vi "Define_Indicies_for_Subtracks_Cost_F()-2.vi"(2 "[IN] Number of Rows":i32, 3 "[IN] Current index":i32, 4 "[IN] Subtracks":T1(array[cluster])) -> (0 "[OUT] Column \n# for Subtrack":i32, 1 "[OUT] Row # \nfor Subtrack":i32)   [LabVIEW 2013]
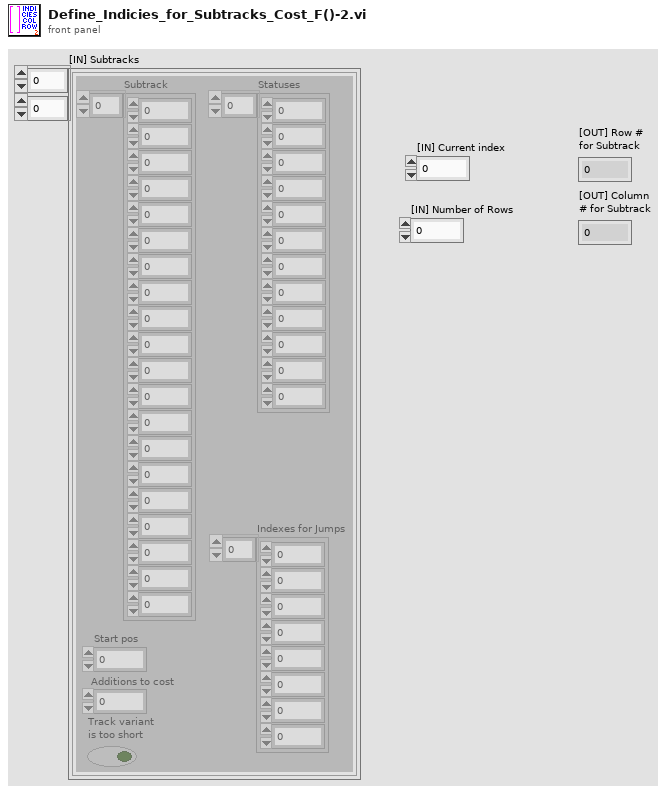
[diagram p1: front panel]
types:
  T1 = cluster{"Subtrack":dbl[], "Statuses":i16[], "Start pos":i32, "Additions to cost":i32, "Track variant \nis too short":bool, "Indexes for Jumps":i32[]}[][]
  T2 = cluster{"Subtrack":dbl[], "Statuses":i16[], "Start pos":i32, "Additions to cost":i32, "Track variant \nis too short":bool, "Indexes for Jumps":i32[]}
  T3 = cluster{"Subtrack":dbl[], "Statuses":i16[], "Start pos":i32, "Additions to cost":i32, "Track variant \nis too short":bool, "Indexes for Jumps":i32[]}[]
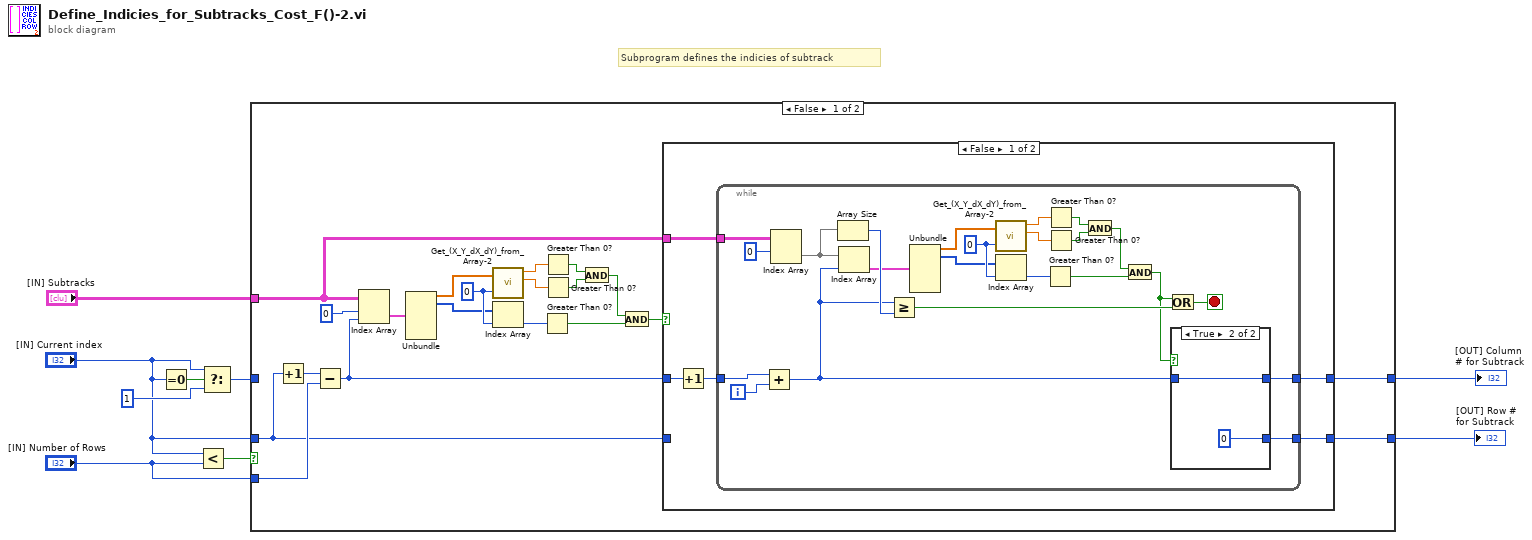
[diagram p0: block diagram]
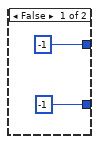
[diagram p2: hidden frame]
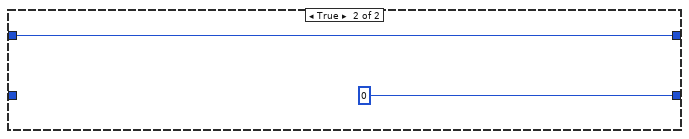
[diagram p3: hidden frame]
diagram:
  # "Subprogram defines the indicies of subtrack"
  n1 = Equal To 0?(x="[IN] Current index") -> (x = 0?=w9:bool)
  n2 = Less?(x="[IN] Current index", y="[IN] Number of Rows") -> (x < y?=w7:bool)
  n3 = Select(t="[IN] Current index", s=w9, f=1) -> (s? t:f=w6:i32)
  n4 = case shown="False" w7 {
    tunnel: w6 -> [_ w65]
    tunnel: [w11 w65] -> w5
    tunnel: "[IN] Current index" -> [w13 w64]
    tunnel: [w12 w64] -> w3
    tunnel: "[IN] Number of Rows" -> [w28 _]
    tunnel: "[IN] Subtracks" -> [w10 _]
    frame False {
      w25 = 0
      n5 = Increment(x=w13) -> (x+1=w29:i32)
      n6 = Subtract(x=w29, y=w28) -> (x-y=w14:i32)
      n7 = Index Array(array=w10, index (row)=0 ("disabled index (row)"), index (col)=w14) -> (element=w26:T2)
      n8 = Unbundle(w26) -> ("Subtrack"=w24:dbl[], "Statuses"=w23:i16[])  [unwired: 4 out]
      n9 = call "Get_(X_Y_dX_dY)_from_Array-2.vi"("(X,Y,dX,dY)"=w24, "Index of Displacement"=w25) -> ("X"=w21:dbl, "Y"=w20:dbl)  [unwired: 2 out]
      n10 = Index Array(array=w23, index=w25) -> (element=w18:i16)
      n11 = Greater Than 0?(x=w18) -> (x > 0?=w16:bool)
      n12 = Greater Than 0?(x=w21) -> (x > 0?=w22:bool)
      n13 = Greater Than 0?(x=w20) -> (x > 0?=w19:bool)
      n14 = And(x=w22, y=w19) -> (x .and. y?=w17:bool)
      n15 = And(x=w17, y=w16) -> (x .and. y?=w15:bool)
      n16 = case shown="False" w15 {
        tunnel: w14 -> [w33 w63]
        tunnel: w13 -> [_ _]
        tunnel: [w30 0 ("[IN] Current index")] -> w12
        tunnel: [w31 w63] -> w11
        tunnel: w10 -> [w34 _]
        frame False {
          n17 = Increment(x=w33) -> (x+1=w32:i32)
          n18 = while {
            tunnel: w34 -> [w57]
            tunnel: w32 -> [w54]
            tunnel: [w36] -> w31
            tunnel: [w35] -> w30
            i -> [w55]
            stop <- w39 stop-if-true
            w51 = 0
            n19 = Add(x=w54, y=w55) -> (x+y=w37:i32)
            n20 = Index Array(array=w57, index (row)=0) -> (element=w53:T3)  [unwired: 1 in]
            n21 = Array Size(array=w53) -> (size(s)=w52:i32)
            n22 = Index Array(array=w53, index=w37) -> (element=w41:T2)
            n23 = Greater Or Equal?(x=w37, y=w52) -> (x >= y?=w40:bool)
            n24 = Unbundle(w41) -> ("Subtrack"=w50:dbl[], "Statuses"=w49:i16[])  [unwired: 4 out]
            n25 = call "Get_(X_Y_dX_dY)_from_Array-2.vi"("(X,Y,dX,dY)"=w50, "Index of Displacement"=w51) -> ("X"=w47:dbl, "Y"=w46:dbl)  [unwired: 2 out]
            n26 = Index Array(array=w49, index=w51) -> (element=w44:i16)
            n27 = Greater Than 0?(x=w44) -> (x > 0?=w42:bool)
            n28 = Greater Than 0?(x=w47) -> (x > 0?=w48:bool)
            n29 = Greater Than 0?(x=w46) -> (x > 0?=w45:bool)
            n30 = And(x=w48, y=w45) -> (x .and. y?=w43:bool)
            n31 = And(x=w43, y=w42) -> (x .and. y?=w38:bool)
            n32 = Or(x=w38, y=w40) -> (x .or. y?=w39:bool)
            n33 = case shown="True" w38 {
              tunnel: w37 -> [_ w61]
              tunnel: [-1 w61] -> w36
              tunnel: [-1 0] -> w35
              frame False {
              }
              frame True {
              }
            }
          }
        }
        frame True {
        }
      }
    }
    frame True {
    }
  }
  "[OUT] Column \n# for Subtrack" <- w5
  "[OUT] Row # \nfor Subtrack" <- w3
